vi "Fetch Measurement(Multiple Points).vi"(0 "VISA resource name":refnum<visa-resource-name>, 5 "Number Of Readings (1)":i32=1, 7 "Timeout Value(10000 ms)":u32=10000, 11 "error in (no error)":errorcluster) -> (4 "VISA resource name out":refnum<visa-resource-name>, 6 "Measurements":sgl[](array[numeric]), 15 "error out":errorcluster)   [LabVIEW 2020, in "3458A Basic Driver.lvlib"]
doc: "Returns an array of values from a previously initiated measurement. The number of measurements the DMM takes is determined by the values you specify for the <B>Trigger Count</B> control of the Read Measurement(Multiple Points) and <B>Sample Count</B> control of the Configure Multipoint VI.\n\n<B>Note:</B> Use this VI only with other low-level VIs. The high-level VIs automatically incorporate this functionality. This VI does not check the instrument status. If you want to check the instrument status, call the Error Query VI at the conclusion of the sequence."
uses:
  3458A Basic Driver.lvlib
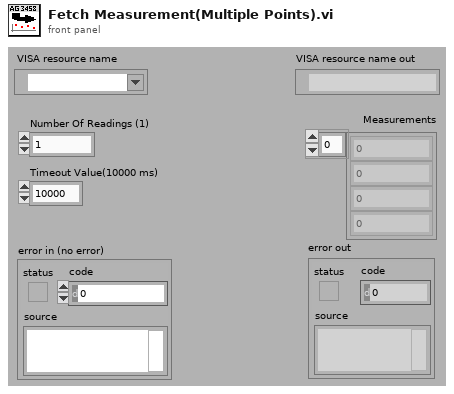
[diagram p1: front panel]
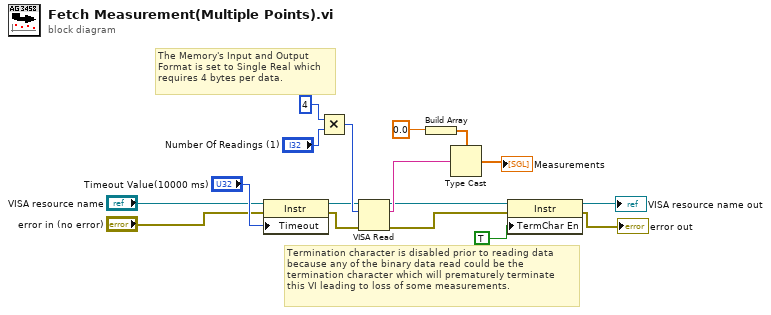
[diagram p0: block diagram]
diagram:
  # "Termination character is disabled prior to reading data\nbecause any of the binary data read could be the \ntermination character which will prematurely terminate\nthis VI leading to loss of some measurements."
  # "The Memory's Input and Output\nFormat is set to Single Real which\nrequires 4 bytes per data."
  n1 = property class="Instr"(reference="VISA resource name", error in="error in (no error)", "Timeout"="Timeout Value(10000 ms)") -> (reference out=w5:refnum<visa-resource-name>, error out=w4:errorcluster)
  n2 = Multiply(x=4, y="Number Of Readings (1)") -> (x*y=w13:i32)
  n3 = VISA Read(VISA resource name=w5, byte count=w13, error in (no error)=w4) -> (VISA resource name out=w12:refnum<visa-resource-name>, read buffer=w14:string, error out=w11:errorcluster)  [unwired: 1 out]
  n4 = Build Array(sgl 0.0) -> (w15:sgl[])
  n5 = Type Cast(type=w15, x=w14) -> (*(type *) &x=→"Measurements":sgl[])
  n6 = property class="Instr"(reference=w12, error in=w11, "TermChar En"=TRUE) -> (reference out=→"VISA resource name out":refnum<visa-resource-name>, error out=→"error out":errorcluster)
